vi "Autonomous Independent.vi"() -> ()   [LabVIEW 2015]
doc: "This VI is called when autonomous begins, and will automatically be terminated when autonomous ends. You can carry out timed or sensor driven robot movement independently without needing to return to the caller."
uses:
  <vilib>/Rock Robotics/WPI/Utilities/WPI_GetSetVariantRefNum.vi
  <vilib>/Rock Robotics/Network Tables/NT Read Number.vi
  Robot Global Data.vi
  <vilib>/Rock Robotics/Network Tables/NT Write Numeric Array.vi
panel:
  in  "F gain":dbl=0.5
  in  "PID Turn gains":T1={"proportional gain (Kc)"=0.008, "integral time (Ti, min)"=0.0, "derivative time (Td, min)"=0.0013}
  in  "Drive Back Speed":dbl=-0.75
  in  "Drive Back Distance":dbl=55.0
  in  "Low Bar Speed":dbl=0.75
  in  "Low Bar Distance":dbl=80.0
  in  "Low Bar Shoot Speed":dbl=0.75
  in  "Low Bar Shoot Distance":dbl=70.0
  in  "CDF Distance 2":dbl=55.0
  in  "CDF Speed 2":dbl=0.75
  out "Scaled Vision X":dbl=-0.010937500000000003
  out "Left Encoder":dbl
  in  "Shoot Bump Distance":dbl=62.0
  in  "Shoot Bump Speed":dbl=1.0
  out "Right Encoder":dbl
  out "Encoder Gyro":dbl
  in  "CDF Distance":dbl=17.0
  in  "CDF Speed":dbl=0.75
  out "Encoder":dbl
  out "Angle":dbl=-9.961713585000021
  in  "Reset Gyro":bool
  in  "Reset Encoder":bool=TRUE
  in  "Bump Speed":dbl=0.75
  in  "Bump Distance":dbl=80.0
  # "Be sure to right-click and choose Data Operations>>Make Current Value default if you want to save the array values with the VI"
  # "THESE ALL DRIVE BACKWARDS\n (towards the tomahawks)\nSet speed to a POSITIVE value"
  # "0 - Do Nothing\n1 - Bump\n2 - CDF \n3 - Low Bar\n4 - Bump Shoot\n5 - CDF Shoot\n6 - Low Bar Shoot\n7 - Spy Shoot"
  # "Spy Auto"
  # "Shoot Autos"
  # "Drive Over Autos"
  # "Bump Shoot"
  # "CDF Shoot"
  # "Low Bar Shoot"
  # "Bump"
  # "CDF"
  # "Low Bar"
  # "Change the arm angle if that doesn't work"
  # "Same Values as don't shoot"
  # "60 now"
  # "Bump Distance 80"
  # "We dont reset this one"
  # "Make add up to bump shoot"
  # "Drive To Middle Zone After Shooting"
  # "This is the one time speed is negative"
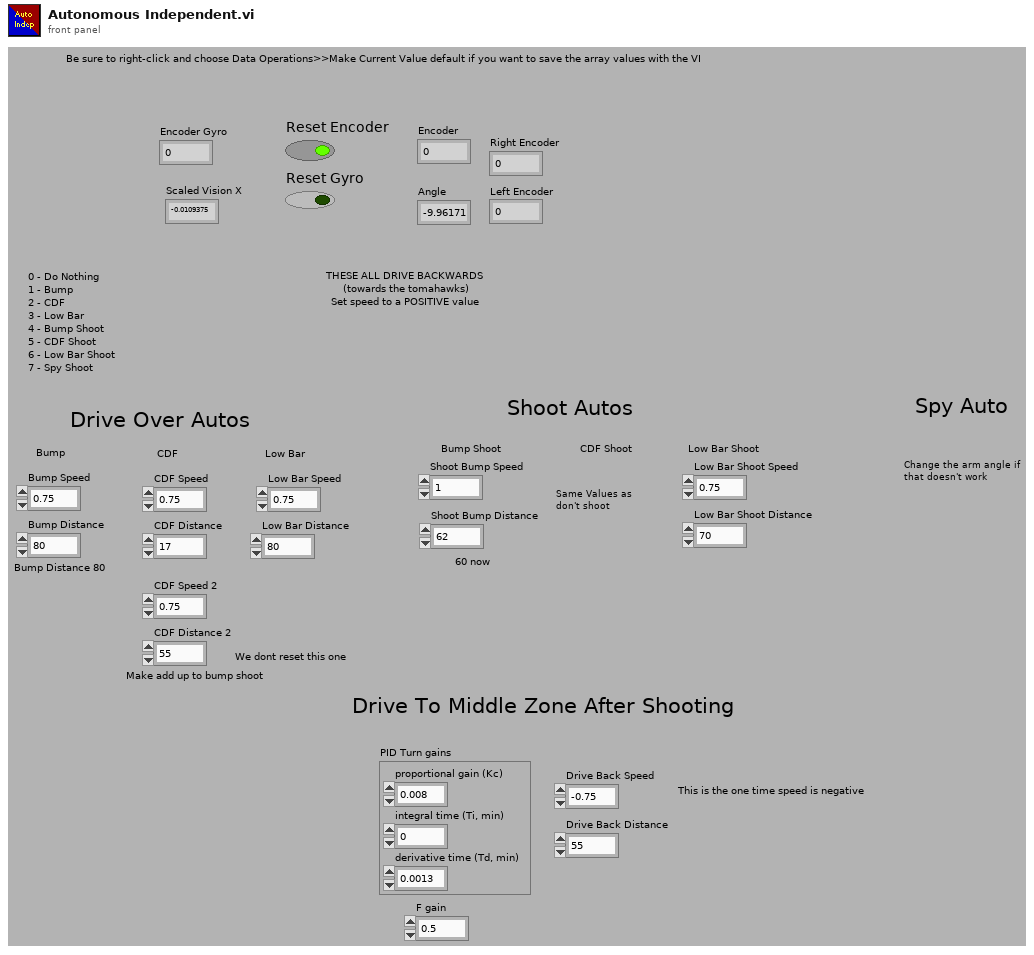
[diagram p1: front panel]
types:
  T1 = cluster{"proportional gain (Kc)":dbl, "integral time (Ti, min)":dbl, "derivative time (Td, min)":dbl}
  T2 = typedef "WPI_JoystickDevRef.ctl" = cluster{"Device":T3}
  T3 = typedef "WPI_JoystickDeviceEnum.ctl" = enum16{"USB 0", "USB 1", "USB 2", "USB 3", "USB 4", "USB 5"}
  T4 = typedef "WPI_GyroDevRef.ctl" = cluster{"DevStatus":errorcluster, "Analog Channel":T5, "Offset":dbl, "Gain (VoltsPerDegree/Second)":dbl, "Gyro Type":enum16{"Analog", "XRS450"}, "Handle":i32, "SPI Bus":T6, "Device Found":bool, "Sample Rate":dbl, "Calibrate On Open":bool}
  T5 = typedef "FPGA_AIChannel.ctl" = enum8{"AI 0", "AI 1", "AI 2", "AI 3", "AI MXP 0", "AI MXP 1", "AI MXP 2", "AI MXP 3", "Invalid"}
  T6 = typedef "spi_bus.ctl" = enum16{"SPI On-Board, CS0", "SPI On-Board, CS1", "SPI On-Board, CS2", "SPI On-Board, CS3", "SPI MXP", "Invalid"}
  T7 = typedef "WPI_EncoderDevRef.ctl" = cluster{"DevStatus":errorcluster, "EncoderIndex":T8, "CounterIndex":T9, "DistancePerCount":dbl, "Decoding Type":T10}
  T8 = typedef "FPGA_EncoderIdx.ctl" = enum8{"Enc 0", "Enc 1", "Enc 2", "Enc 3", "Enc 4", "Enc 5", "Enc 6", "Enc 7", "Invalid"}
  T9 = typedef "FPGA_CounterCtrSystemIndex.ctl" = enum8{"Ctr 0", "Ctr 1", "Ctr 2", "Ctr 3", "Ctr 4", "Ctr 5", "Ctr 6", "Ctr 7", "Invalid"}
  T10 = typedef "WPI_EncoderType.ctl" = enum16{"1x", "2x", "4x"}
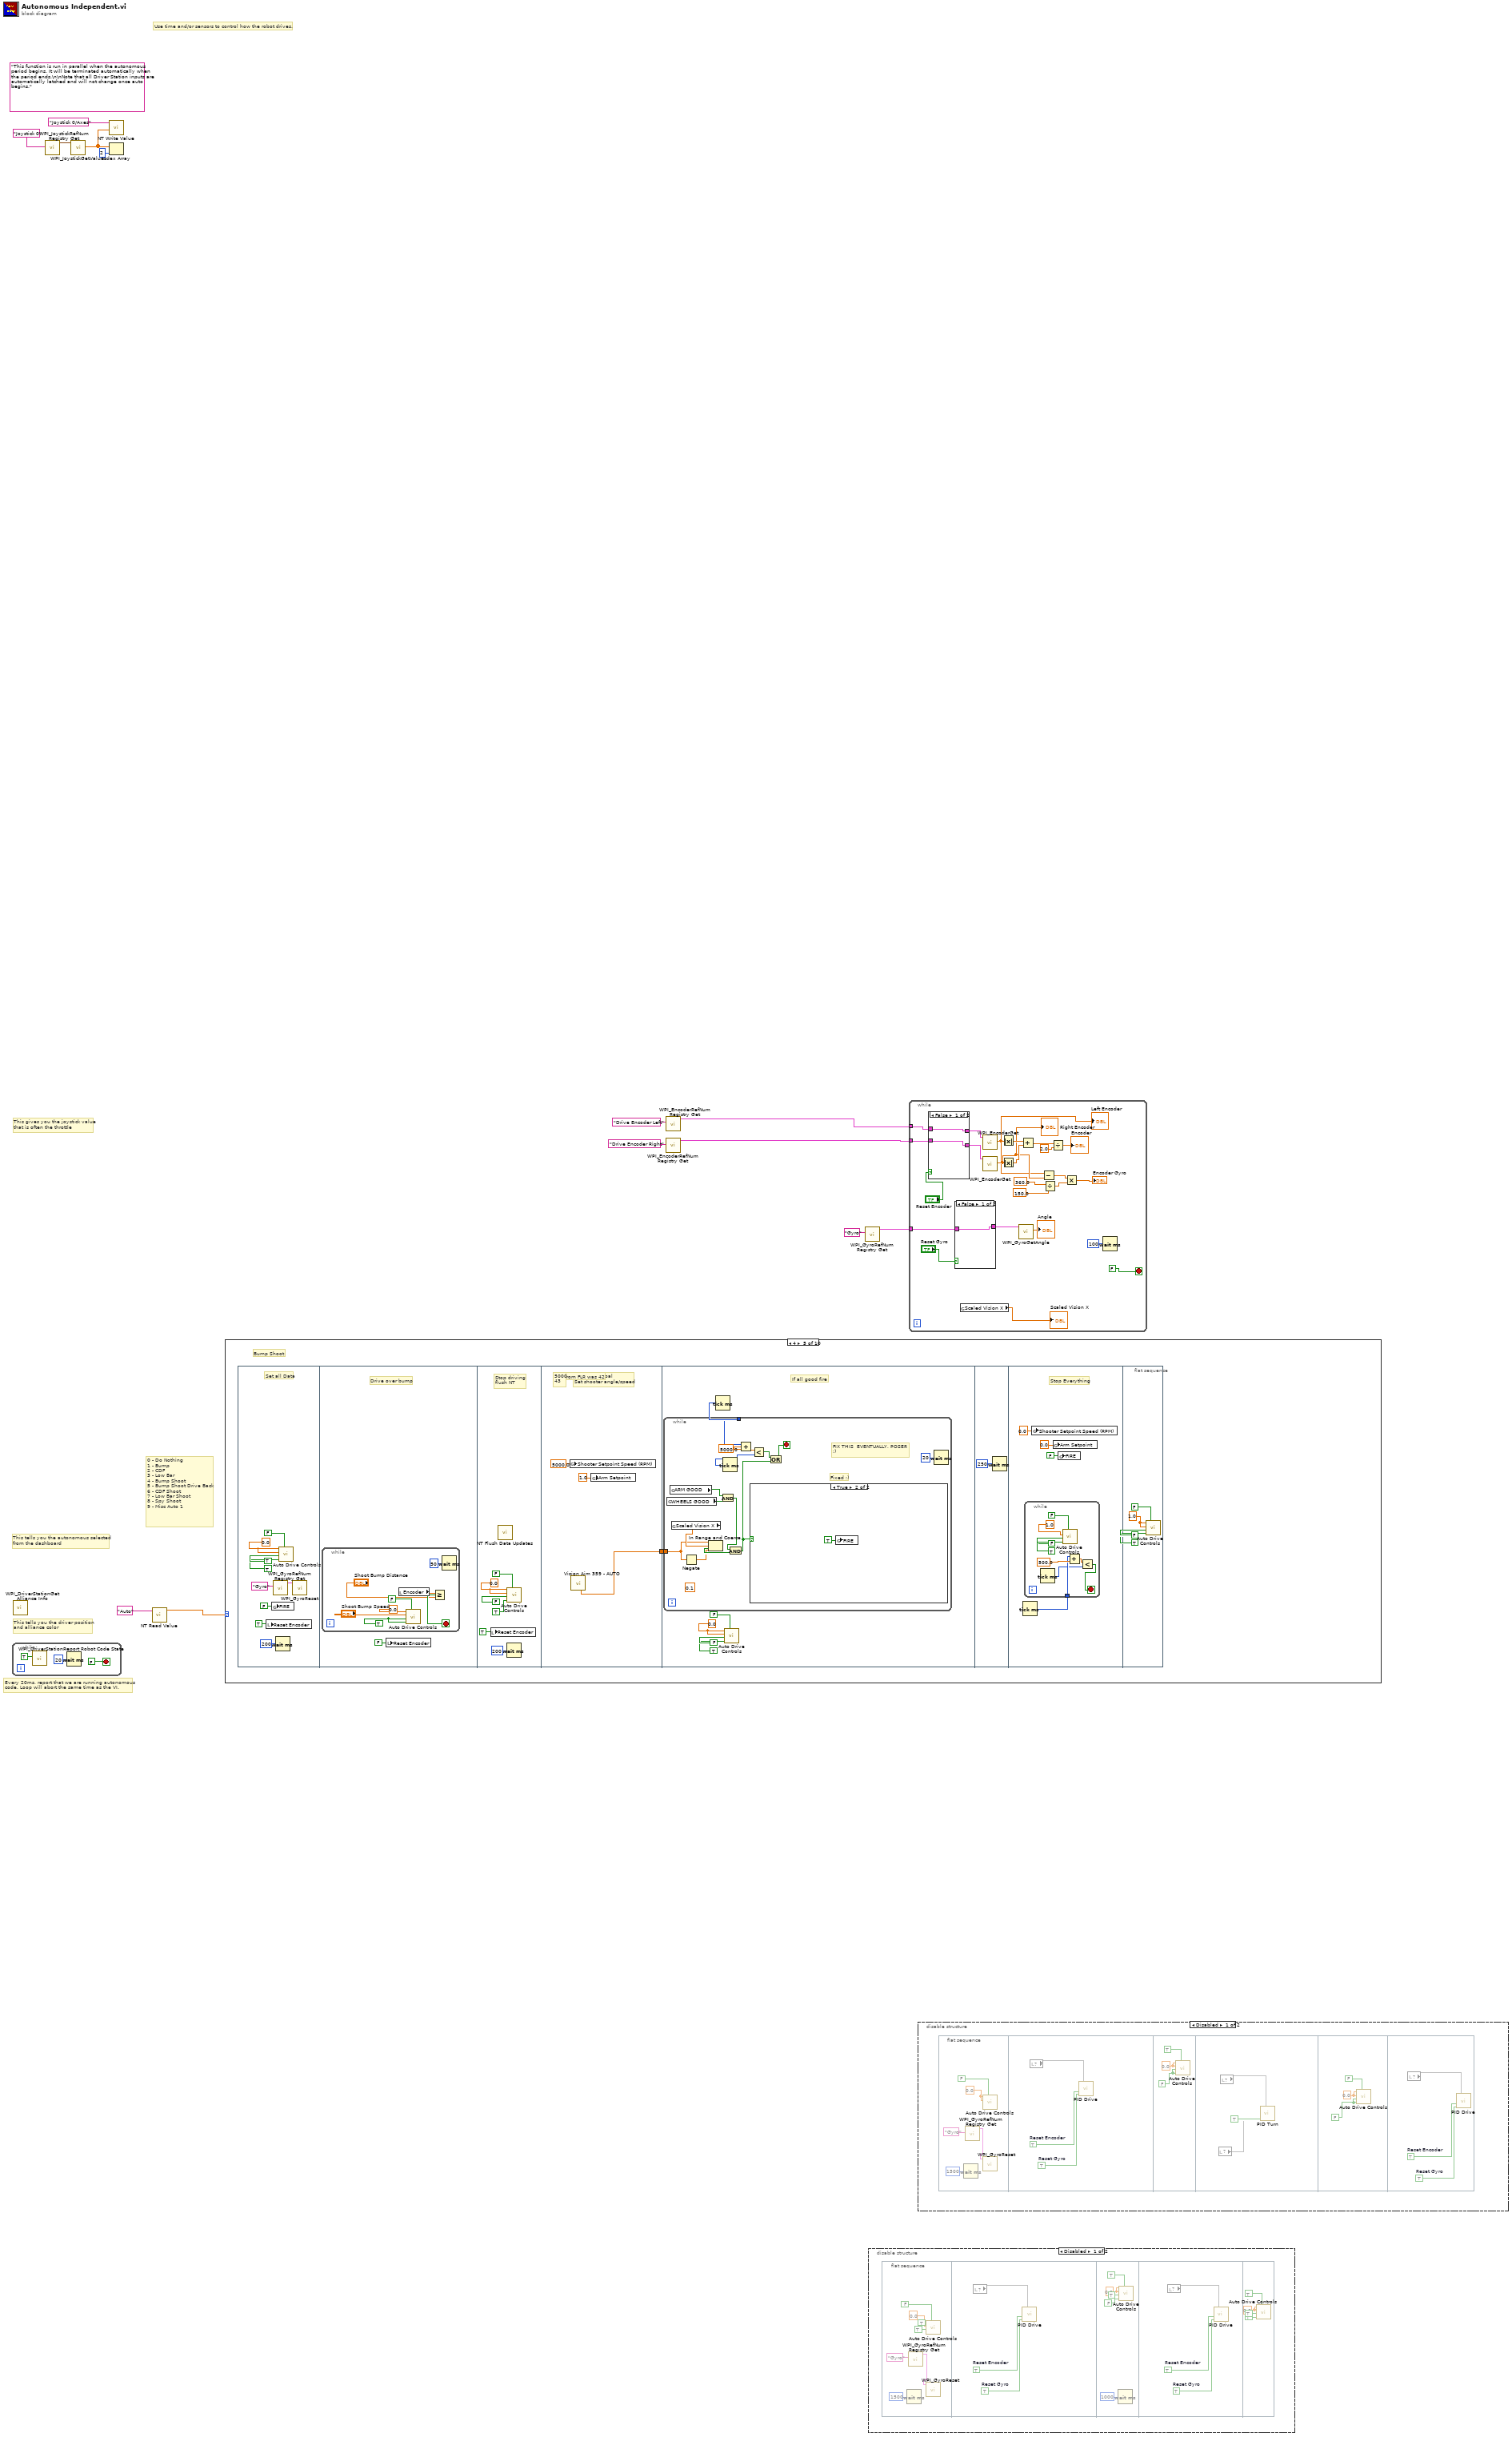
[diagram p0: block diagram]
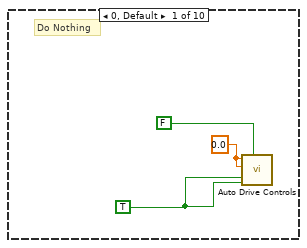
[diagram p2: hidden frame]
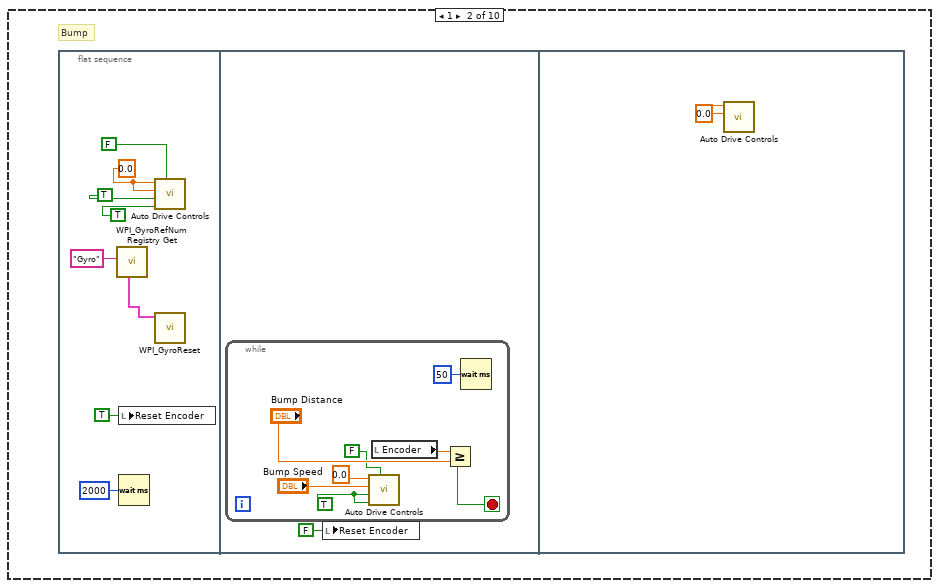
[diagram p3: hidden frame]
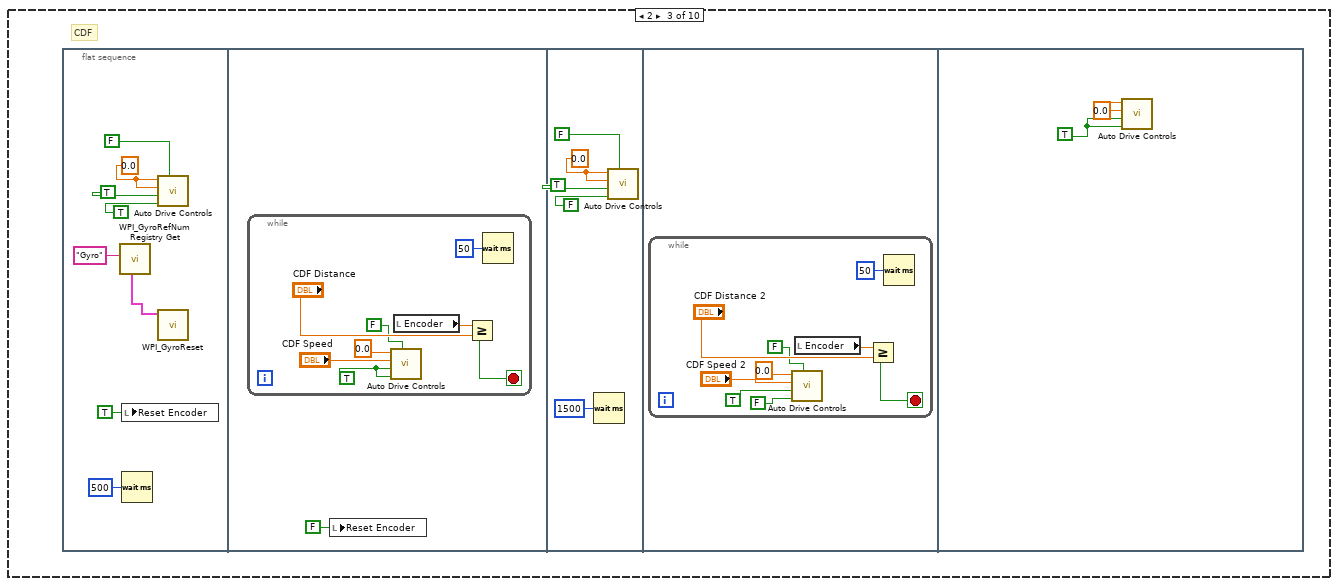
[diagram p4: hidden frame]
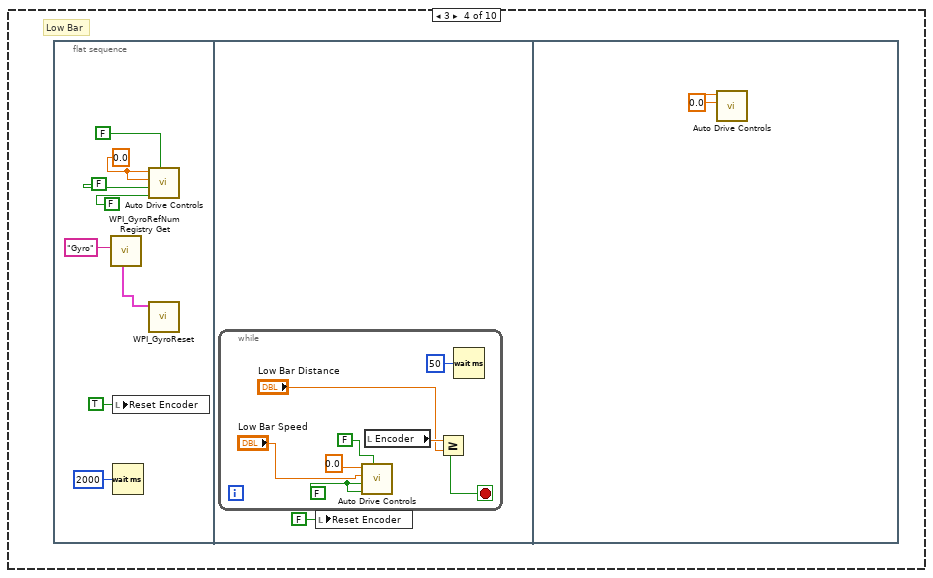
[diagram p5: hidden frame]
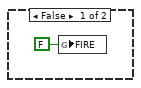
[diagram p6: hidden frame]
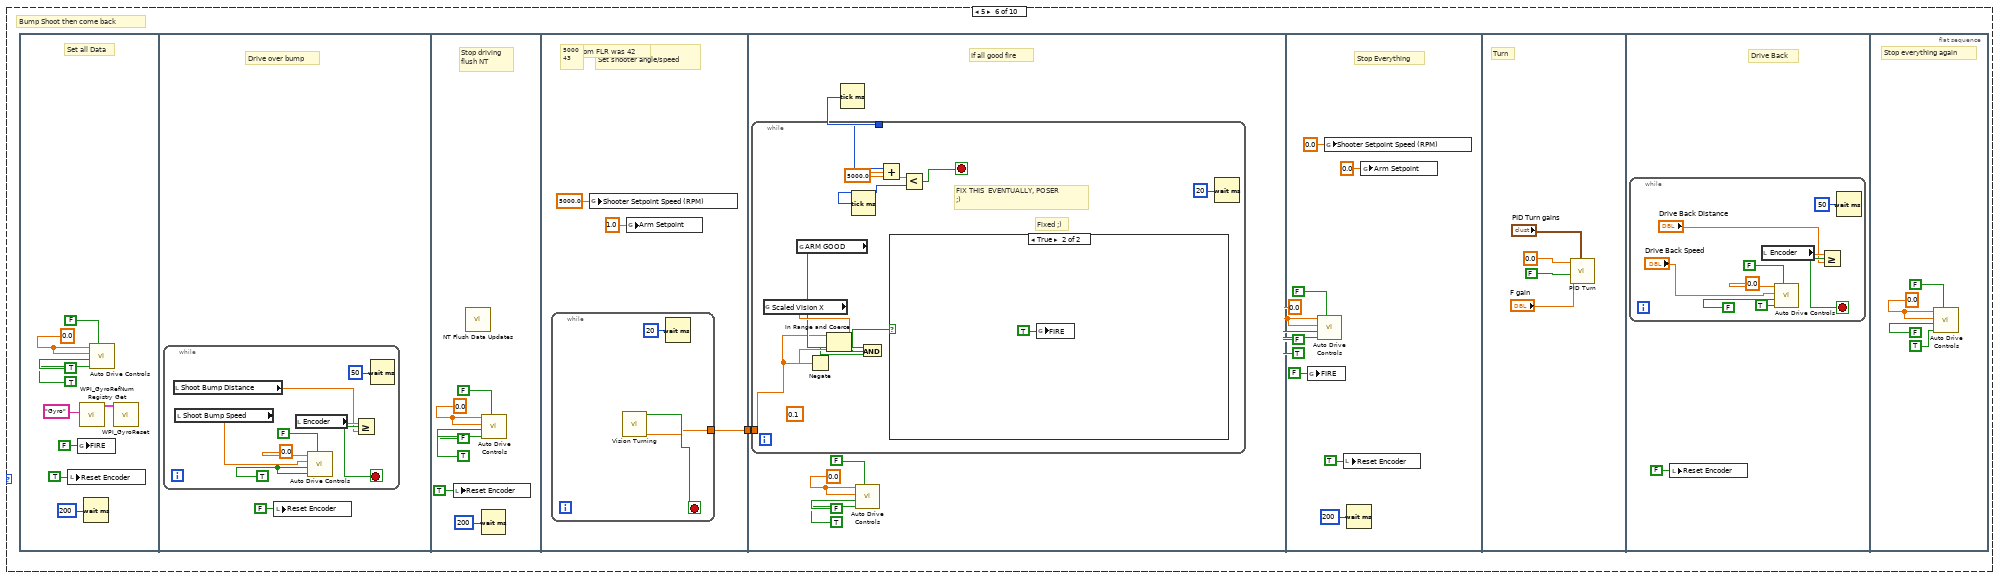
[diagram p7: hidden frame]
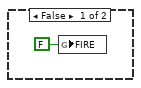
[diagram p8: hidden frame]
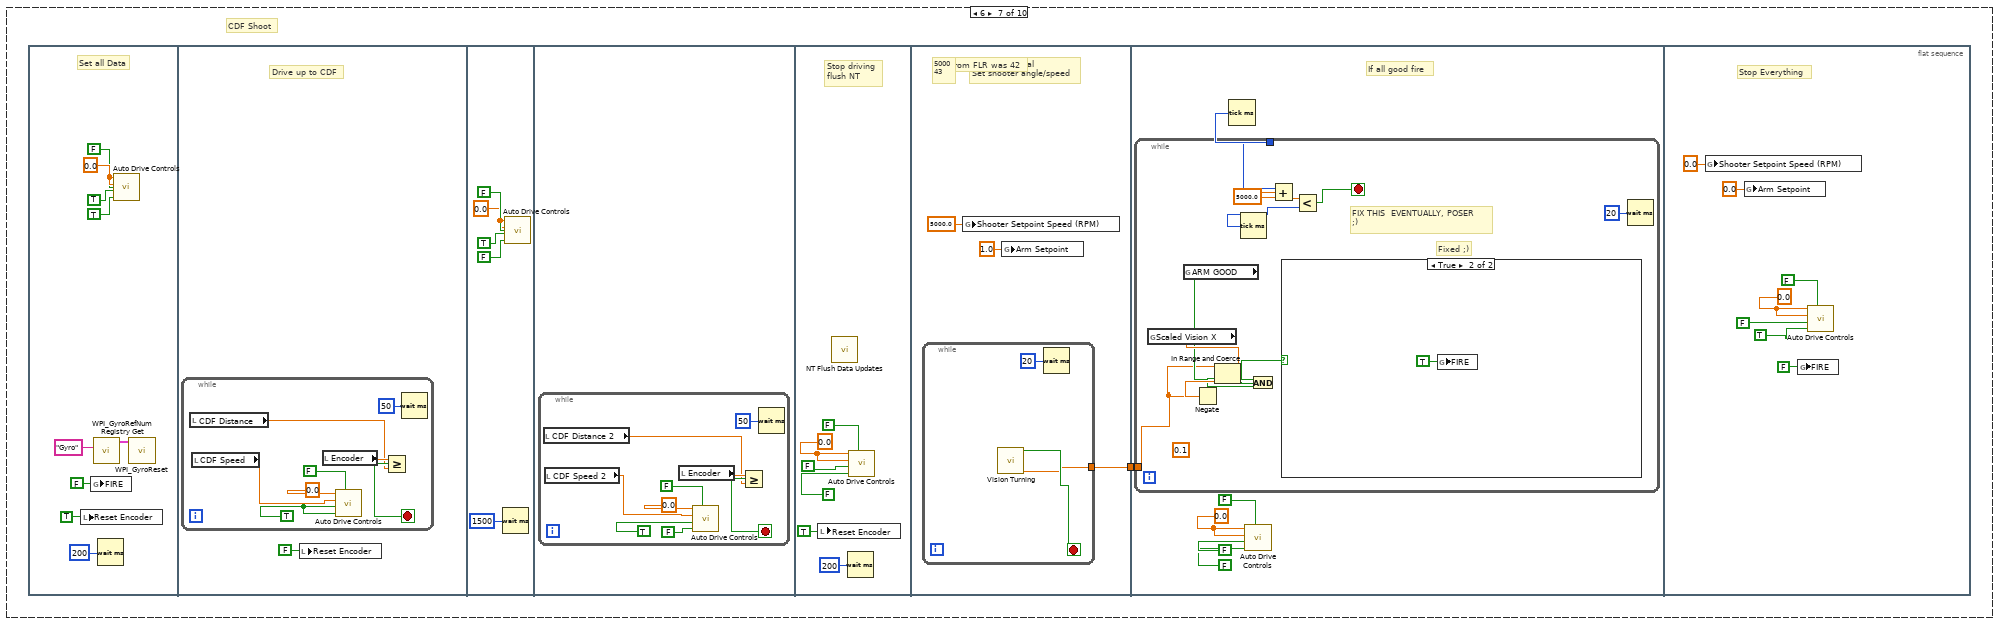
[diagram p9: hidden frame]
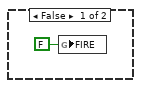
[diagram p10: hidden frame]
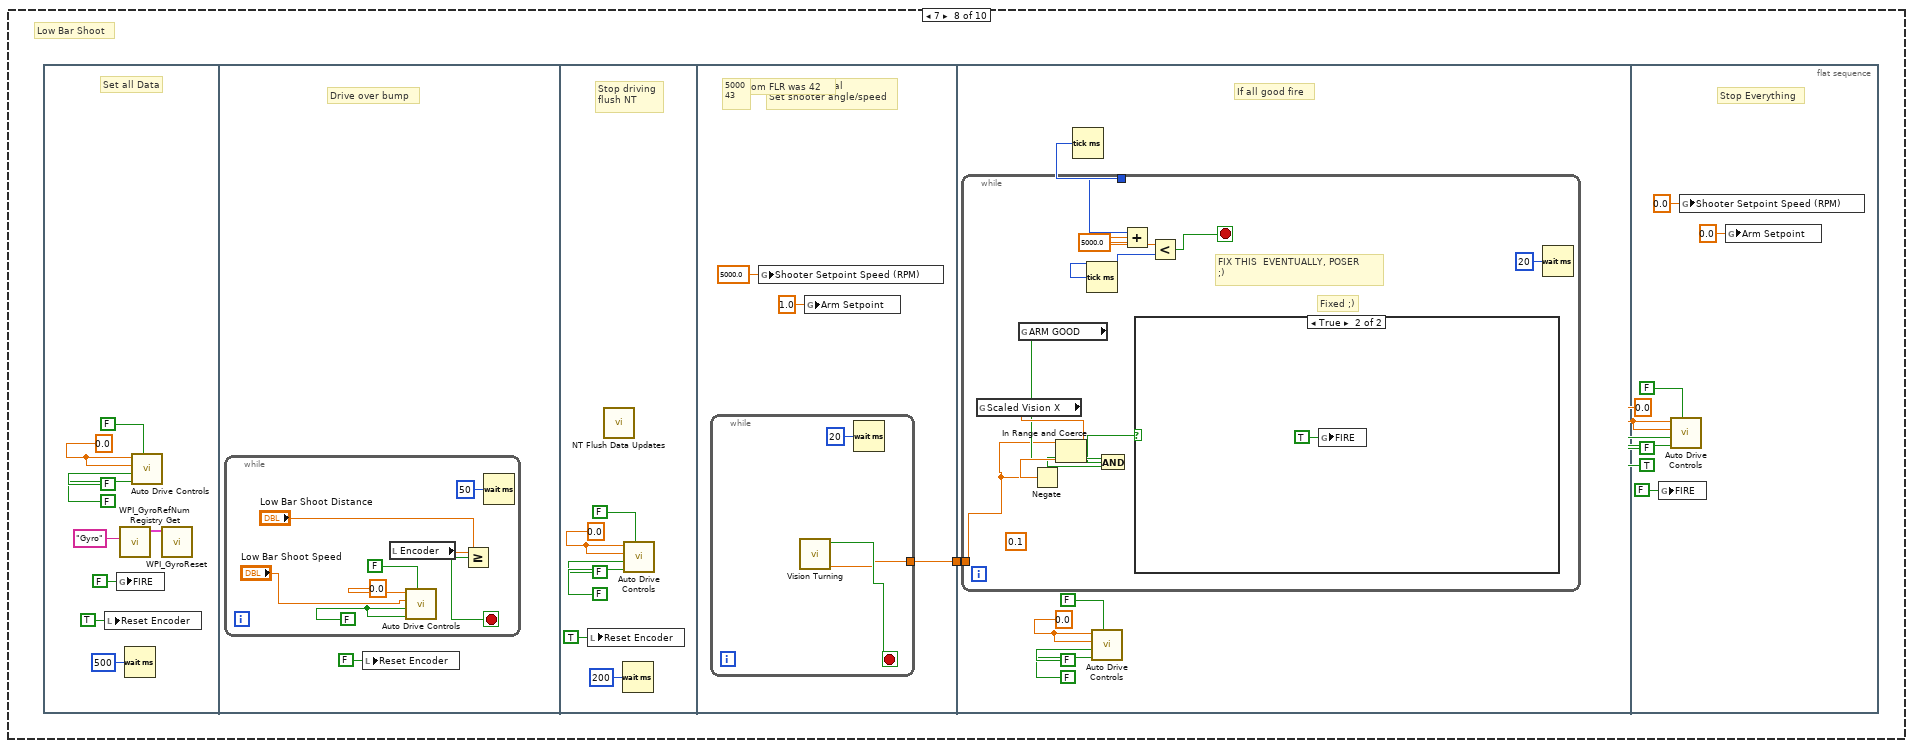
[diagram p11: hidden frame]
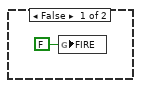
[diagram p12: hidden frame]
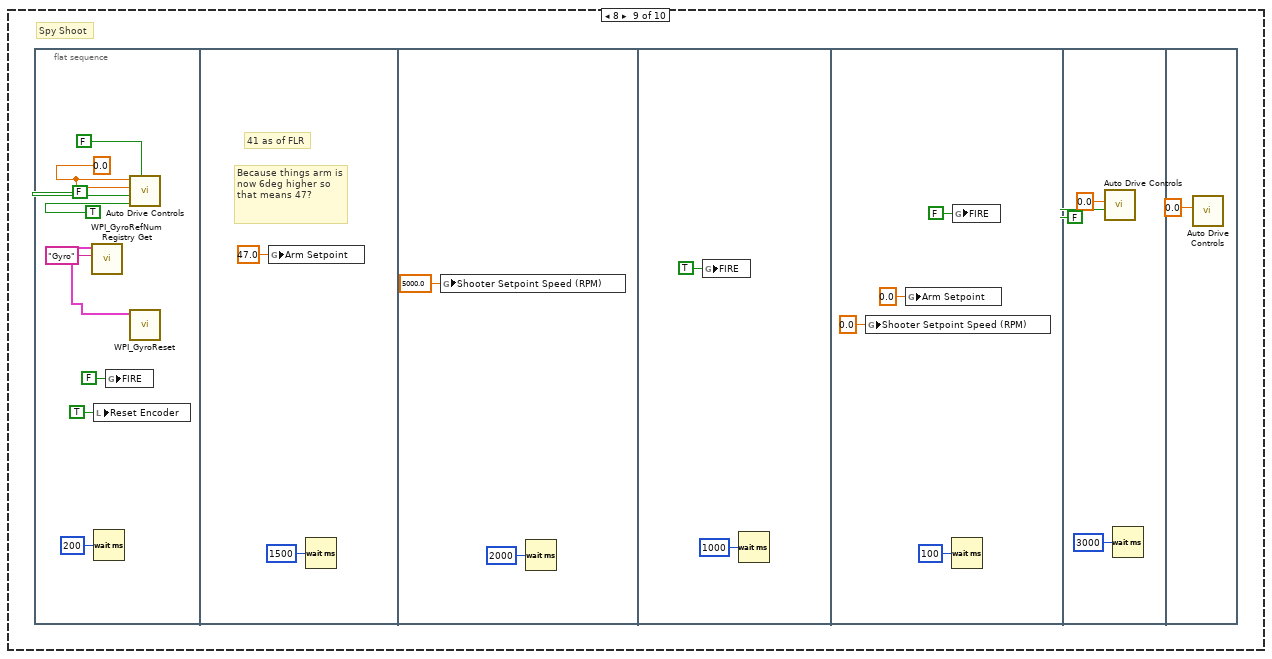
[diagram p13: hidden frame]
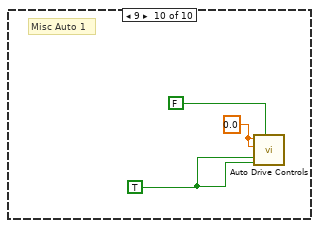
[diagram p14: hidden frame]
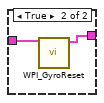
[diagram p17: hidden frame]
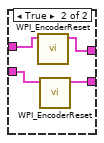
[diagram p18: hidden frame]
diagram:
  (unwired) "This function is run in parallel when the autonomous period begins. It will be terminated automatically when the period ends.\n\nNote that all Driver Station inputs are automatically latched and will not change once auto begins."
  # "0 - Do Nothing\n1 - Bump\n2 - CDF \n3 - Low Bar\n4 - Bump Shoot\n5 - Bump Shoot Drive Back\n6 - CDF Shoot\n7 - Low Bar Shoot\n8 - Spy Shoot\n9 - Misc Auto 1"
  # "This tells you the autonomous selected\nfrom the dashboard"
  # "Every 20ms, report that we are running autonomous\ncode. Loop will abort the same time as the VI."
  # "This gives you the joystick value\nthat is often the throttle"
  # "Use time and/or sensors to control how the robot drives."
  # "This tells you the driver position\nand alliance color"
  n1 = while {
    stop <- FALSE stop-if-true
    n2 = call <vilib>:"WPI_DriverStationReport Robot Code State.vi"("Autonomous"=TRUE) -> ()  [unwired: 10 in, 1 out]
    n3 = Wait (ms)(milliseconds to wait=u32 20) -> ()  [unwired: 1 out]
  }
  n4 = call <vilib>:"WPI_DriverStationGet Alliance Info.vi"() -> ()  [unwired: 12 out]
  n5 = call <vilib>:"WPI_JoystickRefNum Registry Get.vi"("refnum name"="Joystick 0") -> ("JoystickDevRef"=w12:T2)  [unwired: 1 in, 9 out]
  n6 = call <vilib>:"WPI_JoystickGetValues.vi"("JoystickDevRef"=w12) -> ("Axes"=w9:dbl[])  [unwired: 6 in, 4 out]
  n7 = call-poly <vilib>:"NT Write Value.vi"("Numeric Array"=w9, "Name"="Joystick 0/Axes") -> ()  [unwired: 9 in, 1 out]
  n8 = Index Array(array=w9, index=2) -> ()  [unwired: 1 out]
  n9 = call-poly <vilib>:"NT Read Value.vi"("Name"="Auto") -> ("Numeric"=w1:dbl)  [unwired: 9 in, 1 out]
  n10 = case shown="4" w1 {
    frame 0, Default {
      w18 = TRUE ("Intake Up")
      w19 = 0.0 ("X axis value")
      # "Do Nothing"
      n11 = call "Auto Drive Controls.vi"("X axis value"=w19, "Y axis value"=w19, "Intake Up"=w18, "Tomahawk Up"=w18, "Shift High"=FALSE) -> ()  [unwired: 1 in]
    }
    frame 1 {
      # "Bump"
      n12 = flat-sequence {
        frame #0 {
          w27 = 0.0 ("X axis value")
          n13 = call <vilib>:"WPI_GyroRefNum Registry Get.vi"("refnum name"="Gyro") -> ("GyroDevRef"=w24:T4)  [unwired: 9 in, 1 out]
          n14 = local write "Reset Encoder"(TRUE ("Reset Encoder")) -> ()
          n15 = Wait (ms)(milliseconds to wait=u32 2000) -> ()  [unwired: 1 out]
          n16 = call "Auto Drive Controls.vi"("X axis value"=w27, "Y axis value"=w27, "Intake Up"=TRUE, "Tomahawk Up"=TRUE, "Shift High"=FALSE) -> ()  [unwired: 1 in]
          n17 = call <vilib>:"WPI_GyroReset.vi"("GyroDevRef"=w24) -> ()  [unwired: 9 in, 2 out]
        }
        frame #1 {
          n18 = while {
            stop <- w35 stop-if-true
            w30 = TRUE
            n19 = call "Auto Drive Controls.vi"("X axis value"=0.0, "Y axis value"="Bump Speed", "Intake Up"=w30, "Tomahawk Up"=w30, "Shift High"=FALSE) -> ()  [unwired: 1 in]
            n20 = local read "Encoder"() -> (w36:dbl)
            n21 = Greater Or Equal?(x=w36, y="Bump Distance") -> (x >= y?=w35:bool)
            n22 = Wait (ms)(milliseconds to wait=u32 50) -> ()  [unwired: 1 out]
          }
          n23 = local write "Reset Encoder"(FALSE ("Reset Encoder")) -> ()
        }
        frame #2 {
          w37 = 0.0 ("X axis value")
          n24 = call "Auto Drive Controls.vi"("X axis value"=w37, "Y axis value"=w37) -> ()  [unwired: 4 in]
        }
      }
    }
    frame 2 {
      # "CDF"
      n25 = flat-sequence {
        frame #0 {
          w45 = 0.0 ("X axis value")
          n26 = call <vilib>:"WPI_GyroRefNum Registry Get.vi"("refnum name"="Gyro") -> ("GyroDevRef"=w42:T4)  [unwired: 9 in, 1 out]
          n27 = local write "Reset Encoder"(TRUE ("Reset Encoder")) -> ()
          n28 = Wait (ms)(milliseconds to wait=u32 500) -> ()  [unwired: 1 out]
          n29 = call "Auto Drive Controls.vi"("X axis value"=w45, "Y axis value"=w45, "Intake Up"=TRUE, "Tomahawk Up"=TRUE, "Shift High"=FALSE) -> ()  [unwired: 1 in]
          n30 = call <vilib>:"WPI_GyroReset.vi"("GyroDevRef"=w42) -> ()  [unwired: 9 in, 2 out]
        }
        frame #1 {
          n31 = while {
            stop <- w53 stop-if-true
            w48 = TRUE
            n32 = call "Auto Drive Controls.vi"("X axis value"=0.0, "Y axis value"="CDF Speed", "Intake Up"=w48, "Tomahawk Up"=w48, "Shift High"=FALSE) -> ()  [unwired: 1 in]
            n33 = local read "Encoder"() -> (w54:dbl)
            n34 = Greater Or Equal?(x=w54, y="CDF Distance") -> (x >= y?=w53:bool)
            n35 = Wait (ms)(milliseconds to wait=u32 50) -> ()  [unwired: 1 out]
          }
          n36 = local write "Reset Encoder"(FALSE ("Reset Encoder")) -> ()
        }
        frame #2 {
          w56 = 0.0 ("X axis value")
          n37 = Wait (ms)(milliseconds to wait=u32 1500) -> ()  [unwired: 1 out]
          n38 = call "Auto Drive Controls.vi"("X axis value"=w56, "Y axis value"=w56, "Intake Up"=TRUE, "Tomahawk Up"=FALSE, "Shift High"=FALSE) -> ()  [unwired: 1 in]
        }
        frame #3 {
          n39 = while {
            stop <- w67 stop-if-true
            n40 = call "Auto Drive Controls.vi"("X axis value"=0.0, "Y axis value"="CDF Speed 2", "Intake Up"=TRUE, "Tomahawk Up"=FALSE, "Shift High"=FALSE) -> ()  [unwired: 1 in]
            n41 = local read "Encoder"() -> (w68:dbl)
            n42 = Greater Or Equal?(x=w68, y="CDF Distance 2") -> (x >= y?=w67:bool)
            n43 = Wait (ms)(milliseconds to wait=u32 50) -> ()  [unwired: 1 out]
          }
        }
        frame #4 {
          w69 = TRUE ("Intake Up")
          w70 = 0.0 ("X axis value")
          n44 = call "Auto Drive Controls.vi"("X axis value"=w70, "Y axis value"=w70, "Intake Up"=w69, "Tomahawk Up"=w69) -> ()  [unwired: 2 in]
        }
      }
    }
    frame 3 {
      # "Low Bar"
      n45 = flat-sequence {
        frame #0 {
          w78 = 0.0 ("X axis value")
          n46 = call <vilib>:"WPI_GyroRefNum Registry Get.vi"("refnum name"="Gyro") -> ("GyroDevRef"=w75:T4)  [unwired: 9 in, 1 out]
          n47 = local write "Reset Encoder"(TRUE ("Reset Encoder")) -> ()
          n48 = Wait (ms)(milliseconds to wait=u32 2000) -> ()  [unwired: 1 out]
          n49 = call "Auto Drive Controls.vi"("X axis value"=w78, "Y axis value"=w78, "Intake Up"=FALSE, "Tomahawk Up"=FALSE, "Shift High"=FALSE) -> ()  [unwired: 1 in]
          n50 = call <vilib>:"WPI_GyroReset.vi"("GyroDevRef"=w75) -> ()  [unwired: 9 in, 2 out]
        }
        frame #1 {
          n51 = while {
            stop <- w86 stop-if-true
            w83 = FALSE
            n52 = call "Auto Drive Controls.vi"("X axis value"=0.0, "Y axis value"="Low Bar Speed", "Intake Up"=w83, "Tomahawk Up"=w83, "Shift High"=FALSE) -> ()  [unwired: 1 in]
            n53 = local read "Encoder"() -> (w87:dbl)
            n54 = Greater Or Equal?(x=w87, y="Low Bar Distance") -> (x >= y?=w86:bool)
            n55 = Wait (ms)(milliseconds to wait=u32 50) -> ()  [unwired: 1 out]
          }
          n56 = local write "Reset Encoder"(FALSE ("Reset Encoder")) -> ()
        }
        frame #2 {
          w88 = 0.0 ("X axis value")
          n57 = call "Auto Drive Controls.vi"("X axis value"=w88, "Y axis value"=w88) -> ()  [unwired: 4 in]
        }
      }
    }
    frame 4 {
      # "Bump Shoot"
      n58 = flat-sequence {
        tunnel: [w114] -> w89
        tunnel: w89 -> [w117]
        frame #0 {
          w98 = 0.0 ("X axis value")
          # "Set all Data"
          n59 = local write "Reset Encoder"(TRUE ("Reset Encoder")) -> ()
          n60 = global write "Robot Global Data.vi" "FIRE"(FALSE ("FIRE")) -> ()
          n61 = call <vilib>:"WPI_GyroRefNum Registry Get.vi"("refnum name"="Gyro") -> ("GyroDevRef"=w96:T4)  [unwired: 9 in, 1 out]
          n62 = Wait (ms)(milliseconds to wait=u32 200) -> ()  [unwired: 1 out]
          n63 = call "Auto Drive Controls.vi"("X axis value"=w98, "Y axis value"=w98, "Intake Up"=TRUE, "Tomahawk Up"=TRUE, "Shift High"=FALSE) -> ()  [unwired: 1 in]
          n64 = call <vilib>:"WPI_GyroReset.vi"("GyroDevRef"=w96) -> ()  [unwired: 9 in, 2 out]
        }
        frame #1 {
          # "Drive over bump"
          n65 = while {
            stop <- w106 stop-if-true
            w101 = TRUE
            n66 = local read "Encoder"() -> (w107:dbl)
            n67 = call "Auto Drive Controls.vi"("X axis value"=0.0, "Y axis value"="Shoot Bump Speed", "Intake Up"=w101, "Tomahawk Up"=w101, "Shift High"=FALSE) -> ()  [unwired: 1 in]
            n68 = Greater Or Equal?(x=w107, y="Shoot Bump Distance") -> (x >= y?=w106:bool)
            n69 = Wait (ms)(milliseconds to wait=u32 50) -> ()  [unwired: 1 out]
          }
          n70 = local write "Reset Encoder"(FALSE ("Reset Encoder")) -> ()
        }
        frame #2 {
          w108 = 0.0 ("X axis value")
          # "Stop driving\nflush NT"
          n71 = local write "Reset Encoder"(TRUE ("Reset Encoder")) -> ()
          n72 = call <vilib>:"NT Flush Data Updates.vi"() -> ()  [unwired: 11 in, 1 out]
          n73 = Wait (ms)(milliseconds to wait=u32 200) -> ()  [unwired: 1 out]
          n74 = call "Auto Drive Controls.vi"("X axis value"=w108, "Y axis value"=w108, "Intake Up"=FALSE, "Tomahawk Up"=TRUE, "Shift High"=FALSE) -> ()  [unwired: 1 in]
        }
        frame #3 {
          # "Aim at the goal \nSet shooter angle/speed"
          # "5000\n43"
          # "OW from FLR was 42"
          n75 = global write "Robot Global Data.vi" "Shooter Setpoint Speed (RPM)"(5000.0 ("Shooter Setpoint Speed (RPM)")) -> ()
          n76 = call "Vision Aim 359 - AUTO.vi"() -> ("Vision Tolerance  Out"=w114:dbl)  [unwired: 7 in, 4 out]
          n77 = global write "Robot Global Data.vi" "Arm Setpoint"(1.0 ("Arm Setpoint")) -> ()
        }
        frame #4 {
          w122 = 0.0 ("X axis value")
          # "If all good fire"
          n78 = Tick Count (ms)() -> (millisecond timer value=w118:u32)
          n79 = while {
            tunnel: w118 -> [w132]
            tunnel: w117 -> [w129]
            stop <- w124 stop-if-true
            (unwired) 0.1 ("Arm Setpoint")
            # "Fixed ;)"
            # "FIX THIS  EVENTUALLY, POSER \n;)"
            n80 = global read "Robot Global Data.vi" "WHEELS GOOD"() -> (w128:bool)
            n81 = global read "Robot Global Data.vi" "ARM GOOD"() -> (w127:bool)
            n82 = global read "Robot Global Data.vi" "Scaled Vision X"() -> (w137:dbl)
            n83 = Negate(x=w129) -> (-x=w130:dbl)
            n84 = In Range and Coerce(upper limit=w129, x=w137, lower limit=w130) -> (In Range?=w136:bool)  [unwired: 1 out]
            n85 = And(x=w127, y=w128) -> (x .and. y?=w126:bool)
            n86 = Tick Count (ms)() -> (millisecond timer value=w134:u32)
            n87 = And(x=w126, y=w136) -> (x .and. y?=w123:bool)
            n88 = Add(x=w132, y=5000.0) -> (x+y=w133:dbl)
            n89 = case shown="True" w123 {
              frame False {
                n90 = global write "Robot Global Data.vi" "FIRE"(FALSE ("FIRE")) -> ()
              }
              frame True {
                n91 = global write "Robot Global Data.vi" "FIRE"(TRUE ("FIRE")) -> ()
              }
            }
            n92 = Less?(x=w133, y=w134) -> (x < y?=w125:bool)
            n93 = Or(x=w125, y=w123) -> (x .or. y?=w124:bool)
            n94 = Wait (ms)(milliseconds to wait=u32 20) -> ()  [unwired: 1 out]
          }
          n95 = call "Auto Drive Controls.vi"("X axis value"=w122, "Y axis value"=w122, "Intake Up"=FALSE, "Tomahawk Up"=TRUE, "Shift High"=FALSE) -> ()  [unwired: 1 in]
        }
        frame #5 {
          n96 = Wait (ms)(milliseconds to wait=u32 250) -> ()  [unwired: 1 out]
        }
        frame #6 {
          # "Stop Everything"
          n97 = Tick Count (ms)() -> (millisecond timer value=w141:u32)
          n98 = while {
            tunnel: w141 -> [w148]
            stop <- w146 stop-if-true
            n99 = Tick Count (ms)() -> (millisecond timer value=w147:u32)
            n100 = call "Auto Drive Controls.vi"("Y axis value"=1.0 ("X axis value"), "Intake Up"=FALSE, "Tomahawk Up"=TRUE, "Shift High"=FALSE) -> ()  [unwired: 2 in]
            n101 = Add(x=w148, y=500.0) -> (x+y=w150:dbl)
            n102 = Less?(x=w150, y=w147) -> (x < y?=w146:bool)
          }
          n103 = global write "Robot Global Data.vi" "Shooter Setpoint Speed (RPM)"(0.0 ("Shooter Setpoint Speed (RPM)")) -> ()
          n104 = global write "Robot Global Data.vi" "Arm Setpoint"(0.0 ("Arm Setpoint")) -> ()
          n105 = global write "Robot Global Data.vi" "FIRE"(FALSE ("FIRE")) -> ()
        }
        frame #7 {
          w154 = 1.0 ("X axis value")
          n106 = call "Auto Drive Controls.vi"("X axis value"=w154, "Y axis value"=w154, "Intake Up"=FALSE, "Tomahawk Up"=TRUE, "Shift High"=FALSE) -> ()  [unwired: 1 in]
        }
      }
    }
    frame 5 {
      # "Bump Shoot then come back"
      n107 = flat-sequence {
        tunnel: [w183] -> w158
        tunnel: w158 -> [w189]
        frame #0 {
          w167 = 0.0 ("X axis value")
          # "Set all Data"
          n108 = local write "Reset Encoder"(TRUE ("Reset Encoder")) -> ()
          n109 = global write "Robot Global Data.vi" "FIRE"(FALSE ("FIRE")) -> ()
          n110 = call <vilib>:"WPI_GyroRefNum Registry Get.vi"("refnum name"="Gyro") -> ("GyroDevRef"=w165:T4)  [unwired: 9 in, 1 out]
          n111 = Wait (ms)(milliseconds to wait=u32 200) -> ()  [unwired: 1 out]
          n112 = call "Auto Drive Controls.vi"("X axis value"=w167, "Y axis value"=w167, "Intake Up"=TRUE, "Tomahawk Up"=TRUE, "Shift High"=FALSE) -> ()  [unwired: 1 in]
          n113 = call <vilib>:"WPI_GyroReset.vi"("GyroDevRef"=w165) -> ()  [unwired: 9 in, 2 out]
        }
        frame #1 {
          # "Drive over bump"
          n114 = while {
            stop <- w175 stop-if-true
            w172 = TRUE
            n115 = local read "Shoot Bump Distance"() -> (w170:dbl)
            n116 = local read "Shoot Bump Speed"() -> (w169:dbl)
            n117 = local read "Encoder"() -> (w176:dbl)
            n118 = call "Auto Drive Controls.vi"("X axis value"=0.0, "Y axis value"=w169, "Intake Up"=w172, "Tomahawk Up"=w172, "Shift High"=FALSE) -> ()  [unwired: 1 in]
            n119 = Greater Or Equal?(x=w176, y=w170) -> (x >= y?=w175:bool)
            n120 = Wait (ms)(milliseconds to wait=u32 50) -> ()  [unwired: 1 out]
          }
          n121 = local write "Reset Encoder"(FALSE ("Reset Encoder")) -> ()
        }
        frame #2 {
          w177 = 0.0 ("X axis value")
          # "Stop driving\nflush NT"
          n122 = local write "Reset Encoder"(TRUE ("Reset Encoder")) -> ()
          n123 = call <vilib>:"NT Flush Data Updates.vi"() -> ()  [unwired: 11 in, 1 out]
          n124 = Wait (ms)(milliseconds to wait=u32 200) -> ()  [unwired: 1 out]
          n125 = call "Auto Drive Controls.vi"("X axis value"=w177, "Y axis value"=w177, "Intake Up"=FALSE, "Tomahawk Up"=TRUE, "Shift High"=FALSE) -> ()  [unwired: 1 in]
        }
        frame #3 {
          # "Aim at the goal \nSet shooter angle/speed"
          # "5000\n43"
          # "OW from FLR was 42"
          n126 = while {
            tunnel: [w186] -> w183
            stop <- w187 stop-if-true
            n127 = call "Vision Turning.vi"() -> ("Boolean"=w187:bool, "Final Range"=w186:dbl)  [unwired: 6 in, 3 out]
            n128 = Wait (ms)(milliseconds to wait=u32 20) -> ()  [unwired: 1 out]
          }
          n129 = global write "Robot Global Data.vi" "Shooter Setpoint Speed (RPM)"(5000.0 ("Shooter Setpoint Speed (RPM)")) -> ()
          n130 = global write "Robot Global Data.vi" "Arm Setpoint"(1.0 ("Arm Setpoint")) -> ()
        }
        frame #4 {
          w194 = 0.0 ("X axis value")
          # "If all good fire"
          n131 = Tick Count (ms)() -> (millisecond timer value=w190:u32)
          n132 = while {
            tunnel: w190 -> [w198]
            tunnel: w189 -> [w195]
            stop <- w196 stop-if-true
            (unwired) 0.1 ("Arm Setpoint")
            # "Fixed ;)"
            # "FIX THIS  EVENTUALLY, POSER \n;)"
            n133 = global read "Robot Global Data.vi" "Scaled Vision X"() -> (w206:dbl)
            n134 = global read "Robot Global Data.vi" "ARM GOOD"() -> (w203:bool)
            n135 = Negate(x=w195) -> (-x=w205:dbl)
            n136 = In Range and Coerce(upper limit=w195, x=w206, lower limit=w205) -> (In Range?=w204:bool)  [unwired: 1 out]
            n137 = Tick Count (ms)() -> (millisecond timer value=w200:u32)
            n138 = And(x=w203, y=w204) -> (x .and. y?=w202:bool)
            n139 = Add(x=w198, y=5000.0) -> (x+y=w199:dbl)
            n140 = case shown="True" w202 {
              frame False {
                n141 = global write "Robot Global Data.vi" "FIRE"(FALSE ("FIRE")) -> ()
              }
              frame True {
                n142 = global write "Robot Global Data.vi" "FIRE"(TRUE ("FIRE")) -> ()
              }
            }
            n143 = Less?(x=w199, y=w200) -> (x < y?=w196:bool)
            n144 = Wait (ms)(milliseconds to wait=u32 20) -> ()  [unwired: 1 out]
          }
          n145 = call "Auto Drive Controls.vi"("X axis value"=w194, "Y axis value"=w194, "Intake Up"=FALSE, "Tomahawk Up"=TRUE, "Shift High"=FALSE) -> ()  [unwired: 1 in]
        }
        frame #5 {
          w213 = 0.0 ("X axis value")
          # "Stop Everything"
          n146 = global write "Robot Global Data.vi" "FIRE"(FALSE ("FIRE")) -> ()
          n147 = call "Auto Drive Controls.vi"("X axis value"=w213, "Y axis value"=w213, "Intake Up"=FALSE, "Tomahawk Up"=TRUE, "Shift High"=FALSE) -> ()  [unwired: 1 in]
          n148 = global write "Robot Global Data.vi" "Shooter Setpoint Speed (RPM)"(0.0 ("Shooter Setpoint Speed (RPM)")) -> ()
          n149 = local write "Reset Encoder"(TRUE ("Reset Encoder")) -> ()
          n150 = Wait (ms)(milliseconds to wait=u32 200) -> ()  [unwired: 1 out]
          n151 = global write "Robot Global Data.vi" "Arm Setpoint"(0.0 ("Arm Setpoint")) -> ()
        }
        frame #6 {
          # "Turn"
          n152 = call "PID Turn.vi"("PID gains"="PID Turn gains", "F gain"="F gain", "Reset gyro"=FALSE, "Setpoint"=0.0) -> ()  [unwired: 5 in, 3 out]
        }
        frame #7 {
          # "Drive Back"
          n153 = while {
            stop <- w230 stop-if-true
            n154 = local read "Encoder"() -> (w231:dbl)
            n155 = call "Auto Drive Controls.vi"("X axis value"=0.0, "Y axis value"="Drive Back Speed", "Intake Up"=FALSE, "Tomahawk Up"=TRUE, "Shift High"=FALSE) -> ()  [unwired: 1 in]
            n156 = Greater Or Equal?(x=w231, y="Drive Back Distance") -> (x >= y?=w230:bool)
            n157 = Wait (ms)(milliseconds to wait=u32 50) -> ()  [unwired: 1 out]
          }
          n158 = local write "Reset Encoder"(FALSE ("Reset Encoder")) -> ()
        }
        frame #8 {
          w233 = 0.0 ("X axis value")
          # "Stop everything again"
          n159 = call "Auto Drive Controls.vi"("X axis value"=w233, "Y axis value"=w233, "Intake Up"=FALSE, "Tomahawk Up"=TRUE, "Shift High"=FALSE) -> ()  [unwired: 1 in]
        }
      }
    }
    frame 6 {
      # "CDF Shoot"
      n160 = flat-sequence {
        tunnel: [w275] -> w236
        tunnel: w236 -> [w281]
        frame #0 {
          w240 = 0.0 ("X axis value")
          # "Set all Data"
          n161 = local write "Reset Encoder"(TRUE ("Reset Encoder")) -> ()
          n162 = global write "Robot Global Data.vi" "FIRE"(FALSE ("FIRE")) -> ()
          n163 = call <vilib>:"WPI_GyroRefNum Registry Get.vi"("refnum name"="Gyro") -> ("GyroDevRef"=w244:T4)  [unwired: 9 in, 1 out]
          n164 = Wait (ms)(milliseconds to wait=u32 200) -> ()  [unwired: 1 out]
          n165 = call "Auto Drive Controls.vi"("X axis value"=w240, "Y axis value"=w240, "Intake Up"=TRUE, "Tomahawk Up"=TRUE, "Shift High"=FALSE) -> ()  [unwired: 1 in]
          n166 = call <vilib>:"WPI_GyroReset.vi"("GyroDevRef"=w244) -> ()  [unwired: 9 in, 2 out]
        }
        frame #1 {
          # "Drive up to CDF"
          n167 = while {
            stop <- w253 stop-if-true
            w250 = TRUE
            n168 = local read "CDF Distance"() -> (w248:dbl)
            n169 = local read "CDF Speed"() -> (w247:dbl)
            n170 = local read "Encoder"() -> (w254:dbl)
            n171 = call "Auto Drive Controls.vi"("X axis value"=0.0, "Y axis value"=w247, "Intake Up"=w250, "Tomahawk Up"=w250, "Shift High"=FALSE) -> ()  [unwired: 1 in]
            n172 = Greater Or Equal?(x=w254, y=w248) -> (x >= y?=w253:bool)
            n173 = Wait (ms)(milliseconds to wait=u32 50) -> ()  [unwired: 1 out]
          }
          n174 = local write "Reset Encoder"(FALSE ("Reset Encoder")) -> ()
        }
        frame #2 {
          w256 = 0.0 ("X axis value")
          n175 = Wait (ms)(milliseconds to wait=u32 1500) -> ()  [unwired: 1 out]
          n176 = call "Auto Drive Controls.vi"("X axis value"=w256, "Y axis value"=w256, "Intake Up"=TRUE, "Tomahawk Up"=FALSE, "Shift High"=FALSE) -> ()  [unwired: 1 in]
        }
        frame #3 {
          n177 = while {
            stop <- w267 stop-if-true
            n178 = local read "CDF Distance 2"() -> (w262:dbl)
            n179 = local read "CDF Speed 2"() -> (w261:dbl)
            n180 = local read "Encoder"() -> (w268:dbl)
            n181 = call "Auto Drive Controls.vi"("X axis value"=0.0, "Y axis value"=w261, "Intake Up"=TRUE, "Tomahawk Up"=FALSE, "Shift High"=FALSE) -> ()  [unwired: 1 in]
            n182 = Greater Or Equal?(x=w268, y=w262) -> (x >= y?=w267:bool)
            n183 = Wait (ms)(milliseconds to wait=u32 50) -> ()  [unwired: 1 out]
          }
        }
        frame #4 {
          w269 = 0.0 ("X axis value")
          # "Stop driving\nflush NT"
          n184 = local write "Reset Encoder"(TRUE ("Reset Encoder")) -> ()
          n185 = call <vilib>:"NT Flush Data Updates.vi"() -> ()  [unwired: 11 in, 1 out]
          n186 = Wait (ms)(milliseconds to wait=u32 200) -> ()  [unwired: 1 out]
          n187 = call "Auto Drive Controls.vi"("X axis value"=w269, "Y axis value"=w269, "Intake Up"=FALSE, "Tomahawk Up"=FALSE, "Shift High"=FALSE) -> ()  [unwired: 1 in]
        }
        frame #5 {
          # "Aim at the goal \nSet shooter angle/speed"
          # "5000\n43"
          # "OW from FLR was 42"
          n188 = while {
            tunnel: [w278] -> w275
            stop <- w279 stop-if-true
            n189 = call "Vision Turning.vi"() -> ("Boolean"=w279:bool, "Final Range"=w278:dbl)  [unwired: 6 in, 3 out]
            n190 = Wait (ms)(milliseconds to wait=u32 20) -> ()  [unwired: 1 out]
          }
          n191 = global write "Robot Global Data.vi" "Shooter Setpoint Speed (RPM)"(5000.0 ("Shooter Setpoint Speed (RPM)")) -> ()
          n192 = global write "Robot Global Data.vi" "Arm Setpoint"(1.0 ("Arm Setpoint")) -> ()
        }
        frame #6 {
          w286 = 0.0 ("X axis value")
          # "If all good fire"
          n193 = Tick Count (ms)() -> (millisecond timer value=w282:u32)
          n194 = while {
            tunnel: w282 -> [w290]
            tunnel: w281 -> [w287]
            stop <- w288 stop-if-true
            (unwired) 0.1 ("Arm Setpoint")
            # "Fixed ;)"
            # "FIX THIS  EVENTUALLY, POSER \n;)"
            n195 = global read "Robot Global Data.vi" "Scaled Vision X"() -> (w298:dbl)
            n196 = global read "Robot Global Data.vi" "ARM GOOD"() -> (w295:bool)
            n197 = Negate(x=w287) -> (-x=w297:dbl)
            n198 = In Range and Coerce(upper limit=w287, x=w298, lower limit=w297) -> (In Range?=w296:bool)  [unwired: 1 out]
            n199 = Tick Count (ms)() -> (millisecond timer value=w292:u32)
            n200 = And(x=w295, y=w296) -> (x .and. y?=w294:bool)
            n201 = Add(x=w290, y=5000.0) -> (x+y=w291:dbl)
            n202 = case shown="True" w294 {
              frame False {
                n203 = global write "Robot Global Data.vi" "FIRE"(FALSE ("FIRE")) -> ()
              }
              frame True {
                n204 = global write "Robot Global Data.vi" "FIRE"(TRUE ("FIRE")) -> ()
              }
            }
            n205 = Less?(x=w291, y=w292) -> (x < y?=w288:bool)
            n206 = Wait (ms)(milliseconds to wait=u32 20) -> ()  [unwired: 1 out]
          }
          n207 = call "Auto Drive Controls.vi"("X axis value"=w286, "Y axis value"=w286, "Intake Up"=FALSE, "Tomahawk Up"=FALSE, "Shift High"=FALSE) -> ()  [unwired: 1 in]
        }
        frame #7 {
          w301 = 0.0 ("X axis value")
          # "Stop Everything"
          n208 = global write "Robot Global Data.vi" "Shooter Setpoint Speed (RPM)"(0.0 ("Shooter Setpoint Speed (RPM)")) -> ()
          n209 = global write "Robot Global Data.vi" "Arm Setpoint"(0.0 ("Arm Setpoint")) -> ()
          n210 = global write "Robot Global Data.vi" "FIRE"(FALSE ("FIRE")) -> ()
          n211 = call "Auto Drive Controls.vi"("X axis value"=w301, "Y axis value"=w301, "Intake Up"=FALSE, "Tomahawk Up"=TRUE, "Shift High"=FALSE) -> ()  [unwired: 1 in]
        }
      }
    }
    frame 7 {
      # "Low Bar Shoot"
      n212 = flat-sequence {
        tunnel: [w333] -> w308
        tunnel: w308 -> [w339]
        frame #0 {
          w317 = 0.0 ("X axis value")
          # "Set all Data"
          n213 = local write "Reset Encoder"(TRUE ("Reset Encoder")) -> ()
          n214 = global write "Robot Global Data.vi" "FIRE"(FALSE ("FIRE")) -> ()
          n215 = call <vilib>:"WPI_GyroRefNum Registry Get.vi"("refnum name"="Gyro") -> ("GyroDevRef"=w315:T4)  [unwired: 9 in, 1 out]
          n216 = Wait (ms)(milliseconds to wait=u32 500) -> ()  [unwired: 1 out]
          n217 = call "Auto Drive Controls.vi"("X axis value"=w317, "Y axis value"=w317, "Intake Up"=FALSE, "Tomahawk Up"=FALSE, "Shift High"=FALSE) -> ()  [unwired: 1 in]
          n218 = call <vilib>:"WPI_GyroReset.vi"("GyroDevRef"=w315) -> ()  [unwired: 9 in, 2 out]
        }
        frame #1 {
          # "Drive over bump"
          n219 = while {
            stop <- w325 stop-if-true
            w322 = FALSE
            n220 = local read "Encoder"() -> (w326:dbl)
            n221 = call "Auto Drive Controls.vi"("X axis value"=0.0, "Y axis value"="Low Bar Shoot Speed", "Intake Up"=w322, "Tomahawk Up"=w322, "Shift High"=FALSE) -> ()  [unwired: 1 in]
            n222 = Greater Or Equal?(x=w326, y="Low Bar Shoot Distance") -> (x >= y?=w325:bool)
            n223 = Wait (ms)(milliseconds to wait=u32 50) -> ()  [unwired: 1 out]
          }
          n224 = local write "Reset Encoder"(FALSE ("Reset Encoder")) -> ()
        }
        frame #2 {
          w327 = 0.0 ("X axis value")
          # "Stop driving\nflush NT"
          n225 = local write "Reset Encoder"(TRUE ("Reset Encoder")) -> ()
          n226 = call <vilib>:"NT Flush Data Updates.vi"() -> ()  [unwired: 11 in, 1 out]
          n227 = Wait (ms)(milliseconds to wait=u32 200) -> ()  [unwired: 1 out]
          n228 = call "Auto Drive Controls.vi"("X axis value"=w327, "Y axis value"=w327, "Intake Up"=FALSE, "Tomahawk Up"=FALSE, "Shift High"=FALSE) -> ()  [unwired: 1 in]
        }
        frame #3 {
          # "Aim at the goal \nSet shooter angle/speed"
          # "5000\n43"
          # "OW from FLR was 42"
          n229 = while {
            tunnel: [w336] -> w333
            stop <- w337 stop-if-true
            n230 = call "Vision Turning.vi"() -> ("Boolean"=w337:bool, "Final Range"=w336:dbl)  [unwired: 6 in, 3 out]
            n231 = Wait (ms)(milliseconds to wait=u32 20) -> ()  [unwired: 1 out]
          }
          n232 = global write "Robot Global Data.vi" "Shooter Setpoint Speed (RPM)"(5000.0 ("Shooter Setpoint Speed (RPM)")) -> ()
          n233 = global write "Robot Global Data.vi" "Arm Setpoint"(1.0 ("Arm Setpoint")) -> ()
        }
        frame #4 {
          w344 = 0.0 ("X axis value")
          # "If all good fire"
          n234 = Tick Count (ms)() -> (millisecond timer value=w340:u32)
          n235 = while {
            tunnel: w340 -> [w348]
            tunnel: w339 -> [w345]
            stop <- w346 stop-if-true
            (unwired) 0.1 ("Arm Setpoint")
            # "Fixed ;)"
            # "FIX THIS  EVENTUALLY, POSER \n;)"
            n236 = global read "Robot Global Data.vi" "Scaled Vision X"() -> (w356:dbl)
            n237 = global read "Robot Global Data.vi" "ARM GOOD"() -> (w353:bool)
            n238 = Negate(x=w345) -> (-x=w355:dbl)
            n239 = In Range and Coerce(upper limit=w345, x=w356, lower limit=w355) -> (In Range?=w354:bool)  [unwired: 1 out]
            n240 = Tick Count (ms)() -> (millisecond timer value=w350:u32)
            n241 = And(x=w353, y=w354) -> (x .and. y?=w352:bool)
            n242 = Add(x=w348, y=5000.0) -> (x+y=w349:dbl)
            n243 = case shown="True" w352 {
              frame False {
                n244 = global write "Robot Global Data.vi" "FIRE"(FALSE ("FIRE")) -> ()
              }
              frame True {
                n245 = global write "Robot Global Data.vi" "FIRE"(TRUE ("FIRE")) -> ()
              }
            }
            n246 = Less?(x=w349, y=w350) -> (x < y?=w346:bool)
            n247 = Wait (ms)(milliseconds to wait=u32 20) -> ()  [unwired: 1 out]
          }
          n248 = call "Auto Drive Controls.vi"("X axis value"=w344, "Y axis value"=w344, "Intake Up"=FALSE, "Tomahawk Up"=FALSE, "Shift High"=FALSE) -> ()  [unwired: 1 in]
        }
        frame #5 {
          w361 = 0.0 ("X axis value")
          # "Stop Everything"
          n249 = global write "Robot Global Data.vi" "FIRE"(FALSE ("FIRE")) -> ()
          n250 = call "Auto Drive Controls.vi"("X axis value"=w361, "Y axis value"=w361, "Intake Up"=FALSE, "Tomahawk Up"=TRUE, "Shift High"=FALSE) -> ()  [unwired: 1 in]
          n251 = global write "Robot Global Data.vi" "Shooter Setpoint Speed (RPM)"(0.0 ("Shooter Setpoint Speed (RPM)")) -> ()
          n252 = global write "Robot Global Data.vi" "Arm Setpoint"(0.0 ("Arm Setpoint")) -> ()
        }
      }
    }
    frame 8 {
      # "Spy Shoot"
      n253 = flat-sequence {
        frame #0 {
          w374 = 0.0 ("X axis value")
          n254 = call <vilib>:"WPI_GyroRefNum Registry Get.vi"("refnum name"="Gyro") -> ("GyroDevRef"=w371:T4)  [unwired: 9 in, 1 out]
          n255 = local write "Reset Encoder"(TRUE ("Reset Encoder")) -> ()
          n256 = Wait (ms)(milliseconds to wait=u32 200) -> ()  [unwired: 1 out]
          n257 = global write "Robot Global Data.vi" "FIRE"(FALSE ("FIRE")) -> ()
          n258 = call "Auto Drive Controls.vi"("X axis value"=w374, "Y axis value"=w374, "Intake Up"=FALSE, "Tomahawk Up"=TRUE, "Shift High"=FALSE) -> ()  [unwired: 1 in]
          n259 = call <vilib>:"WPI_GyroReset.vi"("GyroDevRef"=w371) -> ()  [unwired: 9 in, 2 out]
        }
        frame #1 {
          # "Because things arm is now 6deg higher so that means 47?"
          # "41 as of FLR"
          n260 = global write "Robot Global Data.vi" "Arm Setpoint"(47.0 ("Arm Setpoint")) -> ()
          n261 = Wait (ms)(milliseconds to wait=u32 1500) -> ()  [unwired: 1 out]
        }
        frame #2 {
          n262 = global write "Robot Global Data.vi" "Shooter Setpoint Speed (RPM)"(5000.0 ("Shooter Setpoint Speed (RPM)")) -> ()
          n263 = Wait (ms)(milliseconds to wait=u32 2000) -> ()  [unwired: 1 out]
        }
        frame #3 {
          n264 = global write "Robot Global Data.vi" "FIRE"(TRUE ("FIRE")) -> ()
          n265 = Wait (ms)(milliseconds to wait=u32 1000) -> ()  [unwired: 1 out]
        }
        frame #4 {
          n266 = global write "Robot Global Data.vi" "Shooter Setpoint Speed (RPM)"(0.0 ("Shooter Setpoint Speed (RPM)")) -> ()
          n267 = global write "Robot Global Data.vi" "Arm Setpoint"(0.0 ("Arm Setpoint")) -> ()
          n268 = Wait (ms)(milliseconds to wait=u32 100) -> ()  [unwired: 1 out]
          n269 = global write "Robot Global Data.vi" "FIRE"(FALSE ("FIRE")) -> ()
        }
        frame #5 {
          n270 = call "Auto Drive Controls.vi"("Y axis value"=0.0 ("X axis value"), "Intake Up"=FALSE) -> ()  [unwired: 4 in]
          n271 = Wait (ms)(milliseconds to wait=u32 3000) -> ()  [unwired: 1 out]
        }
        frame #6 {
          n272 = call "Auto Drive Controls.vi"("Y axis value"=0.0 ("X axis value")) -> ()  [unwired: 5 in]
        }
      }
    }
    frame 9 {
      w390 = TRUE ("Intake Up")
      w391 = 0.0 ("X axis value")
      # "Misc Auto 1"
      n273 = call "Auto Drive Controls.vi"("X axis value"=w391, "Y axis value"=w391, "Intake Up"=w390, "Tomahawk Up"=w390, "Shift High"=FALSE) -> ()  [unwired: 1 in]
    }
  }
  n274 = call <vilib>:"WPI_EncoderRefNum Registry Get.vi"("refnum name"="Drive Encoder Left") -> ("EncoderDevRef"=w3:T7)  [unwired: 9 in, 1 out]
  n275 = call <vilib>:"WPI_EncoderRefNum Registry Get.vi"("refnum name"="Drive Encoder Right") -> ("EncoderDevRef"=w4:T7)  [unwired: 9 in, 1 out]
  n276 = call <vilib>:"WPI_GyroRefNum Registry Get.vi"("refnum name"="Gyro") -> ("GyroDevRef"=w2:T4)  [unwired: 9 in, 1 out]
  n277 = disable-structure shown="Disabled" {
    frame Disabled {
      n278 = flat-sequence {
        frame #0 {
          w398 = 0.0 ("X axis value")
          n279 = Wait (ms)(milliseconds to wait=u32 1500) -> ()  [unwired: 1 out]
          n280 = call <vilib>:"WPI_GyroRefNum Registry Get.vi"("refnum name"="Gyro") -> ("GyroDevRef"=w395:T4)  [unwired: 9 in, 1 out]
          n281 = call "Auto Drive Controls.vi"("X axis value"=w398, "Y axis value"=w398, "Intake Up"=TRUE, "Tomahawk Up"=TRUE, "Shift High"=FALSE) -> ()  [unwired: 1 in]
          n282 = call <vilib>:"WPI_GyroReset.vi"("GyroDevRef"=w395) -> ()  [unwired: 9 in, 2 out]
        }
        frame #1 {
          w402 = TRUE  # Reset Gyro
          w403 = TRUE  # Reset Encoder
          n283 = local read item#-1() -> (w399)
          n284 = call "PID Drive.vi"("PID gains"=w399, "Reset Encoder"=w403, "Reset Gyro"=w402) -> ("Setpoint Distance"=w401:dbl, "Speed"=w400:dbl)  [unwired: 9 in, 2 out]
        }
        frame #2 {
          w408 = 0.0 ("X axis value")
          n285 = Wait (ms)(milliseconds to wait=u32 1000) -> ()  [unwired: 1 out]
          n286 = call "Auto Drive Controls.vi"("X axis value"=w408, "Y axis value"=w408, "Intake Up"=TRUE, "Tomahawk Up"=FALSE, "Shift High"=TRUE) -> ()  [unwired: 1 in]
        }
        frame #3 {
          w411 = TRUE  # Reset Gyro
          w410 = TRUE  # Reset Encoder
          n287 = local read item#-1() -> (w409)
          n288 = call "PID Drive.vi"("PID gains"=w409, "Reset Encoder"=w410, "Reset Gyro"=w411) -> ("Setpoint Distance"=w412:dbl, "Speed"=w413:dbl)  [unwired: 9 in, 2 out]
        }
        frame #4 {
          w416 = 0.0 ("X axis value")
          n289 = call "Auto Drive Controls.vi"("X axis value"=w416, "Y axis value"=w416, "Intake Up"=TRUE, "Tomahawk Up"=TRUE, "Shift High"=TRUE) -> ()  [unwired: 1 in]
        }
      }
    }
    frame Enabled {
    }
  }
  n290 = while {
    tunnel: w4 -> [w431]
    tunnel: w3 -> [w432]
    tunnel: w2 -> [w428]
    stop <- FALSE stop-if-true
    n291 = case shown="False" "Reset Encoder" {
      tunnel: [w446 w450] -> w429
      tunnel: [w445 w449] -> w430
      tunnel: w432 -> [w446 w448]
      tunnel: w431 -> [w445 w447]
      frame False {
      }
      frame True {
        n292 = call <vilib>:"WPI_EncoderReset.vi"("EncoderDevRef"=w448) -> ("EncoderDevRef"=w450:T7)  [unwired: 9 in, 1 out]
        n293 = call <vilib>:"WPI_EncoderReset.vi"("EncoderDevRef"=w447) -> ("EncoderDevRef"=w449:T7)  [unwired: 9 in, 1 out]
      }
    }
    n294 = case shown="False" "Reset Gyro" {
      tunnel: [w442 w444] -> w427
      tunnel: w428 -> [w442 w443]
      frame False {
      }
      frame True {
        n295 = call <vilib>:"WPI_GyroReset.vi"("GyroDevRef"=w443) -> ("GyroDevRef"=w444:T4)  [unwired: 9 in, 1 out]
      }
    }
    n296 = global read "Robot Global Data.vi" "Scaled Vision X"() -> (→"Scaled Vision X":dbl)
    n297 = call <vilib>:"WPI_EncoderGet.vi"("EncoderDevRef"=w429) -> ("Distance"=w419:dbl)  [unwired: 5 in, 5 out]
    "Left Encoder" <- w419
    n298 = call <vilib>:"WPI_EncoderGet.vi"("EncoderDevRef"=w430) -> ("Distance"=w420:dbl)  [unwired: 5 in, 5 out]
    "Right Encoder" <- w420
    n299 = Absolute Value(x=w419) -> (abs(x)=w439:dbl)
    n300 = Absolute Value(x=w420) -> (abs(x)=w438:dbl)
    n301 = call <vilib>:"WPI_GyroGetAngle.vi"("GyroDevRef"=w427) -> ("Angle"=→"Angle":dbl)  [unwired: 6 in, 4 out]
    n302 = Add(x=w439, y=w438) -> (x+y=w441:dbl)
    n303 = Subtract(x=w419, y=w420) -> (x-y=w425:dbl)
    n304 = Divide(x=360.0, y=150.0) -> (x/y=w423:dbl)
    n305 = Divide(x=w441, y=2.0) -> (x/y=→"Encoder":dbl)
    n306 = Multiply(x=w425, y=w423) -> (x*y=→"Encoder Gyro":dbl)
    n307 = Wait (ms)(milliseconds to wait=u32 100) -> ()  [unwired: 1 out]
  }
  n308 = disable-structure shown="Disabled" {
    frame Disabled {
      n309 = flat-sequence {
        frame #0 {
          w457 = 0.0 ("X axis value")
          n310 = Wait (ms)(milliseconds to wait=u32 1500) -> ()  [unwired: 1 out]
          n311 = call <vilib>:"WPI_GyroRefNum Registry Get.vi"("refnum name"="Gyro") -> ("GyroDevRef"=w454:T4)  [unwired: 9 in, 1 out]
          n312 = call "Auto Drive Controls.vi"("X axis value"=w457, "Y axis value"=w457, "Shift High"=FALSE) -> ("Intake Up"=w452:bool, "Tomahawk Up"=w451:bool)  [unwired: 1 in]
          n313 = call <vilib>:"WPI_GyroReset.vi"("GyroDevRef"=w454) -> ()  [unwired: 9 in, 2 out]
        }
        frame #1 {
          w461 = TRUE  # Reset Gyro
          w462 = TRUE  # Reset Encoder
          n314 = local read item#-1() -> (w458)
          n315 = call "PID Drive.vi"("PID gains"=w458, "Reset Encoder"=w462, "Reset Gyro"=w461) -> ("Setpoint Distance"=w460:dbl, "Speed"=w459:dbl)  [unwired: 9 in, 2 out]
        }
        frame #2 {
          w463 = FALSE ("Shift High")
          w465 = 0.0 ("X axis value")
          n316 = call "Auto Drive Controls.vi"("X axis value"=w465, "Y axis value"=w465, "Intake Up"=w463, "Tomahawk Up"=w463, "Shift High"=TRUE) -> ()  [unwired: 1 in]
        }
        frame #3 {
          n317 = local read item#-1() -> (w466)
          n318 = local read item#-1() -> (w467)
          n319 = call "PID Turn.vi"("PID gains"=w467, "F gain"=w466, "Reset gyro"=TRUE) -> ("Setpoint"=w468:dbl)  [unwired: 5 in, 3 out]
        }
        frame #4 {
          w470 = FALSE ("Shift High")
          w472 = 0.0 ("X axis value")
          n320 = call "Auto Drive Controls.vi"("X axis value"=w472, "Y axis value"=w472, "Intake Up"=w470, "Tomahawk Up"=w470, "Shift High"=FALSE) -> ()  [unwired: 1 in]
        }
        frame #5 {
          w474 = TRUE  # Reset Gyro
          w473 = TRUE  # Reset Encoder
          n321 = local read item#-1() -> (w477)
          n322 = call "PID Drive.vi"("PID gains"=w477, "Reset Encoder"=w473, "Reset Gyro"=w474) -> ("Setpoint Distance"=w475:dbl, "Speed"=w476:dbl)  [unwired: 9 in, 2 out]
        }
      }
    }
    frame Enabled {
    }
  }
